vi "QDMH Launch.vi"(8 "error in (no error)":errorcluster, 9 "Front Panel Window (Open)":bool, 10 "Queue Name":string, 11 "VI Path":path) -> (0 "error out":errorcluster, 3 "Launched VI Name":string)   [LabVIEW 2011]
doc: "This VI will launch a dynamic process. \n\nAAL 9/09"
uses:
  <vilib>/Utility/traverseref.llb/TRef TravTarget.ctl
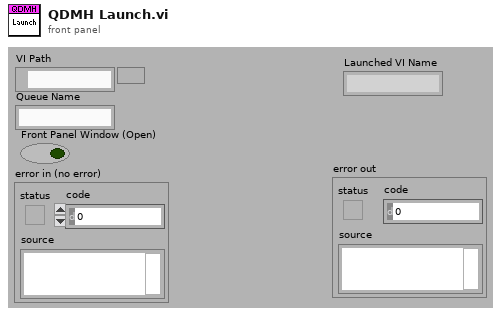
[diagram p1: front panel]
types:
  T1 = typedef "TRef TravTarget.ctl" = enum16{"FP", "BD", "Other"}
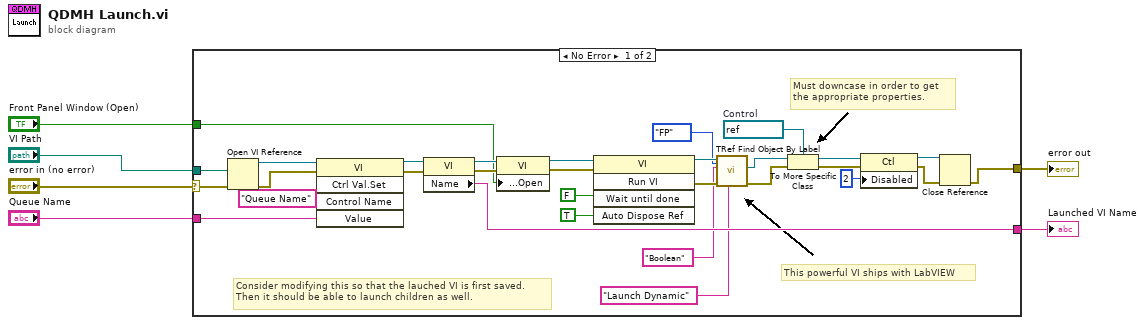
[diagram p0: block diagram]
diagram:
  n1 = case shown="No Error" "error in (no error)" {
    selector: "error in (no error)" -> [w22 w38]
    tunnel: "Queue Name" -> [w36 w37]
    tunnel: [w9 w38] -> w5
    tunnel: [w30 w37] -> w4
    tunnel: "VI Path" -> [w28 _]
    tunnel: "Front Panel Window (Open)" -> [w23 _]
    frame No Error {
      w14 = refnum<vi> refnum  # Control
      # "Must downcase in order to get\nthe appropriate properties."
      # "This powerful VI ships with LabVIEW"
      # "Consider modifying this so that the lauched VI is first saved.\nThen it should be able to launch children as well."
      n2 = Open VI Reference(vi path=w28, error in (no error)=w22) -> (vi reference=w21:refnum<vi>, error out=w32:errorcluster)  [unwired: 4 out]
      n3 = invoke class="VI" method="Ctrl Val.Set"(reference=w21, error in=w32, "Control Name"="Queue Name", "Value"=w36) -> (reference out=w33:refnum<vi>, error out=w34:errorcluster)  [unwired: 1 in, 3 out]
      n4 = property class="VI"(reference=w33, error in=w34) -> (reference out=w29:refnum<vi>, error out=w31:errorcluster, "Name"=w30:string)
      n5 = property class="VI"(reference=w29, error in=w31, "Front Panel.Open"=w23) -> (reference out=w25:refnum<vi>, error out=w24:errorcluster)
      n6 = invoke class="VI" method="Run VI"(reference=w25, error in=w24, "Wait until done"=FALSE ("Wait Until Done"), "Auto Dispose Ref"=TRUE ("Auto Dispose Reference")) -> (reference out=w19:refnum<vi>, error out=w18:errorcluster)  [unwired: 1 in, 3 out]
      n7 = call <vilib>:"TRef Find Object By Label.vi"("Label"="Launch Dynamic", "Traverse Target"=TRef_TravTarget."FP", "error in (no error)"=w18, "Class Name"="Boolean", "VI Ref"=w19) -> ("error out"=w16:errorcluster, "Found Obj Ref"=w17:refnum<vi>)  [unwired: 1 in, 4 out]
      n8 = To More Specific Class(target class=w14, reference=w17, error in=w16) -> (specific class reference=w13:refnum<vi>, error out=w15:errorcluster)
      n9 = property class="Ctl"(reference=w13, error in=w15, "Disabled"=u8 2) -> (reference out=w10:refnum<vi>, error out=w11:errorcluster)
      n10 = Close Reference(reference=w10, error in (no error)=w11) -> (error out=w9:errorcluster)
    }
    frame Error {
    }
  }
  "error out" <- w5
  "Launched VI Name" <- w4
